vi "MIMO Plant Simulator.vi"(0 "Initial PV":dbl[](array[numeric]) format="%.2f", 1 "dt (s)":dbl=-1.0 format="%.3f", 2 "Measurement Noise (%)":dbl(slide) scale=0.0..100.0, 4 "Controller Noise (%)":dbl(slide) scale=0.0..100.0, 5 "Valve Deadband":dbl format="%.1f", 6 "Process Deadtime":i32(slide) scale=0.0..5.0, 7 "Lags":dbl[](array[numeric]) format="%.2f", 8 "Plant Load":dbl[](array[slide]) scale=0.0..5.0, 9 "Plant Gains":dbl[](array[slide]) scale=0.0..5.0, 10 "Manipulated Variable (MV)":dbl[](array[numeric]) format="%.2f", 11 "iteration":i32) -> (3 "Process Variable":dbl[](array[numeric]) format="%.2f")   [LabVIEW 2023]
doc: "Simulates a physical plant's response; for use with feedback control loops.\n\nAll scale factors are in percent. Lag time is in minutes. Process Deadtime is a true deadtime, measured as a multiple of the loop cycle time. NOTE: this deadtime is dependent upon the interval at which this VI is called. You can modify the algorithm used here to simulate almost any process.\n\nIf more than one plant needs to be simulated simultaneously, save multiple copies of this VI under different names."
uses:
  <vilib>/addons/control/pid/pid.llb/PID Lead-Lag (DBL Array).vi
  <vilib>/addons/control/pid/NI_PID_pid.lvlib
panel:
  # "Plant Characteristics"
  # "(x cycle time)"
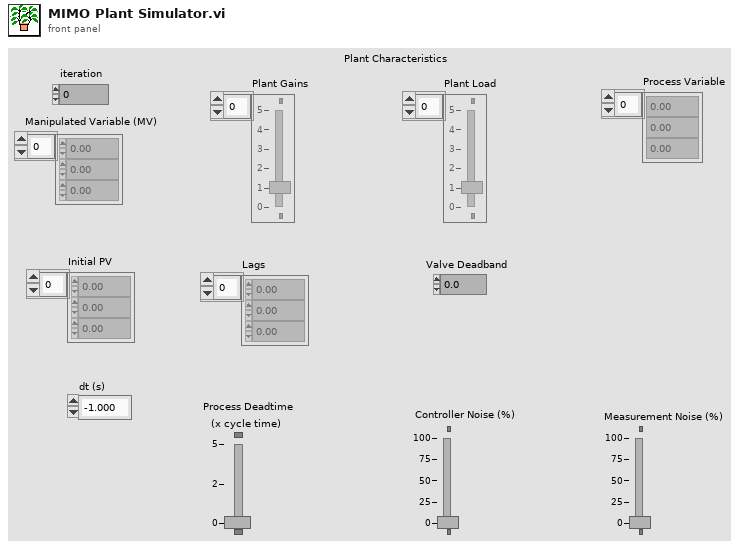
[diagram p1: front panel]
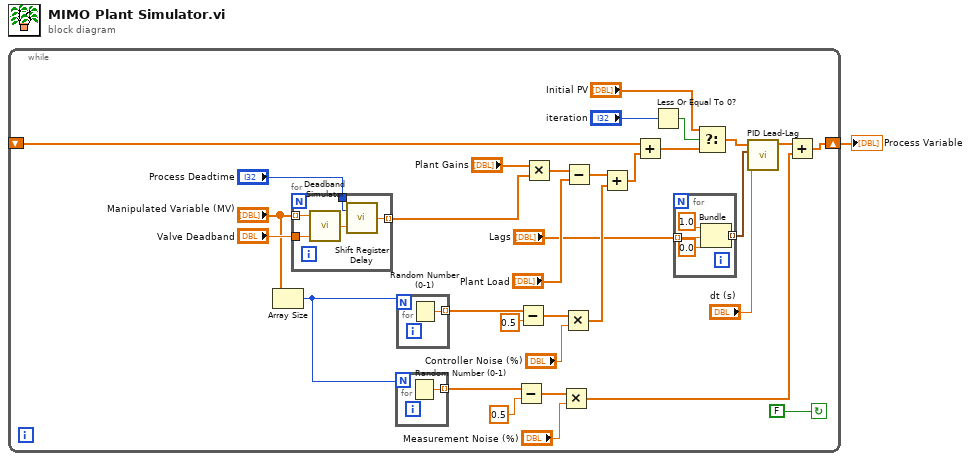
[diagram p0: block diagram]
diagram:
  n1 = while {
    shift-left: _ -> [w15]
    shift-right: [w9] -> w1
    stop <- FALSE continue-if-true
    n2 = Array Size(array="Manipulated Variable (MV)") -> (size(s)=w4:i32)
    n3 = for {
      tunnel: "Valve Deadband" -> [w39]
      tunnel: "Manipulated Variable (MV)" -> [w38] mode=indexing
      tunnel: [w37] -> w31 mode=indexing
      tunnel: "Process Deadtime" -> [w36]
      n4 = call "Deadband Simulator.vi"("deadband (%)"=w39, "requested pos. (%)"=w38) -> ("actual pos. (%)"=w40:dbl)  [unwired: 1 in]
      n5 = call "Shift Register Delay.vi"("input"=w40, "n delay (0)"=w36) -> ("output"=w37:dbl)
    }
    n6 = for {
      N: w4 -> [_]
      tunnel: [w34] -> w2 mode=indexing
      n7 = Random Number (0-1)() -> (number: 0 to 1=w34:dbl)
    }
    n8 = for {
      N: w4 -> [_]
      tunnel: [w35] -> w3 mode=indexing
      n9 = Random Number (0-1)() -> (number: 0 to 1=w35:dbl)
    }
    n10 = Subtract(x=w2, y=0.5) -> (x-y=w12:dbl[])
    n11 = Subtract(x=w3, y=0.5) -> (x-y=w28:dbl[])
    n12 = Multiply(x="Plant Gains", y=w31) -> (x*y=w23:dbl[])
    n13 = Multiply(x=w12, y="Measurement Noise (%)") -> (x*y=w8:dbl[])
    n14 = Multiply(x=w28, y="Controller Noise (%)") -> (x*y=w33:dbl[])
    n15 = Subtract(x=w23, y="Plant Load") -> (x-y=w24:dbl[])
    n16 = Add(x=w24, y=w33) -> (x+y=w27:dbl[])
    n17 = Add(x=w15, y=w27) -> (x+y=w22:dbl[])
    n18 = Less Or Equal To 0?(x="iteration") -> (x <= 0?=w20:bool)
    n19 = for {
      tunnel: [w44] -> w17 mode=indexing
      tunnel: "Lags" -> [w43] mode=indexing
      n20 = Bundle(1.0, "Lag (min)"=w43, 0.0) -> (w44:cluster{dbl, "Lag (min)":dbl, dbl})  [unwired: 1 in]
    }
    n21 = Select(t="Initial PV", s=w20, f=w22) -> (s? t:f=w21:dbl[])
    n22 = call-poly <vilib>:"PID Lead-Lag.vi"("dt (s)"="dt (s)", "tuning parameters"=w17, "input"=w21) -> ("output"=w10:dbl[])  [unwired: 5 in, 1 out]
    n23 = Add(x=w10, y=w8) -> (x+y=w9:dbl[])
  }
  "Process Variable" <- w1
